vi "Error parser.vi"(0 "Data Readed":string, 11 "error in (no error)":errorcluster) -> (15 "error out":errorcluster)   [LabVIEW 2024, in "GRBL 1.1.lvlib"]
doc: "This Vi transfort error status from GRBL to LabVIEW inteligible error code."
uses:
  GRBL 1.1.lvlib
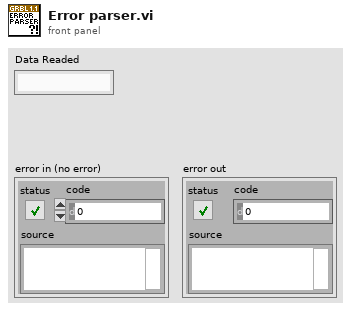
[diagram p1: front panel]
types:
  T1 = cluster{"Code V1.1":i32, "error constant":errorcluster}[]
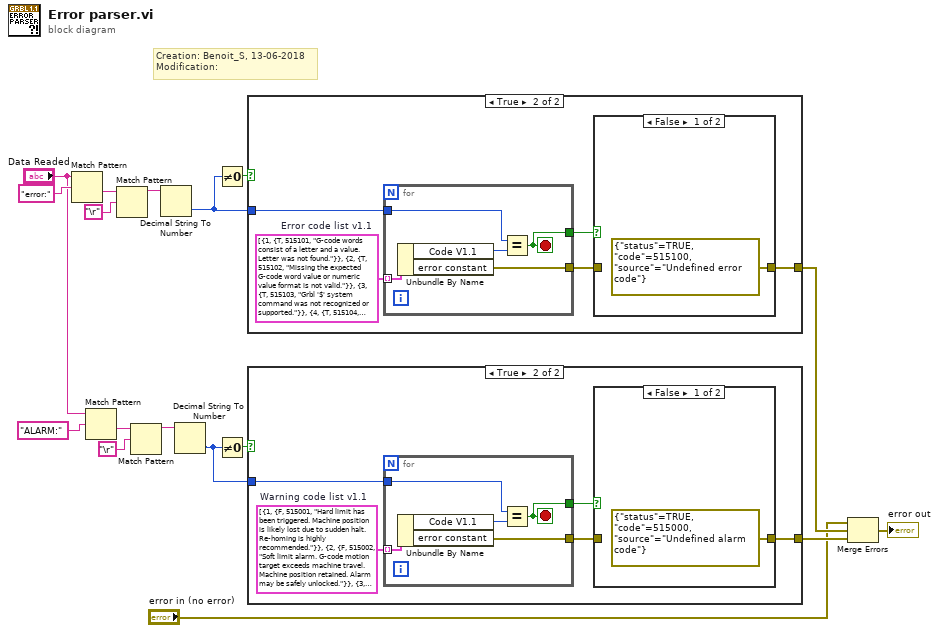
[diagram p0: block diagram]
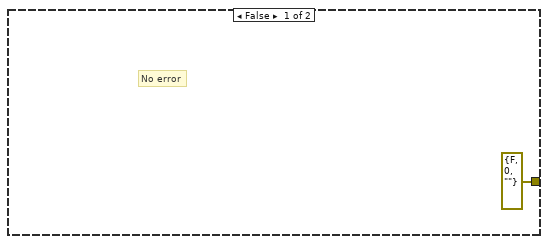
[diagram p2: hidden frame]
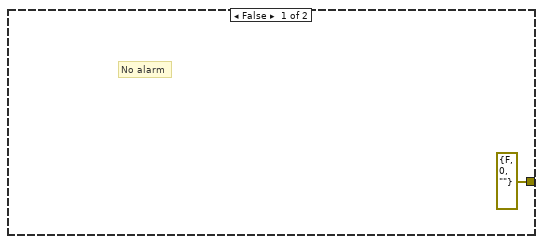
[diagram p4: hidden frame]
diagram:
  # "Creation: Benoit_S, 13-06-2018\nModification:"
  n1 = Match Pattern(string="Data Readed", regular expression="error:") -> (after substring=w10:string)  [unwired: 1 in, 3 out]
  n2 = Match Pattern(string="Data Readed", regular expression="ALARM:") -> (after substring=w4:string)  [unwired: 1 in, 3 out]
  n3 = Match Pattern(string=w10, regular expression="\r") -> (before substring=w8:string)  [unwired: 1 in, 3 out]
  n4 = Match Pattern(string=w4, regular expression="\r") -> (before substring=w6:string)  [unwired: 1 in, 3 out]
  n5 = Decimal String To Number(string=w8) -> (number=w7:i32)  [unwired: 2 in, 1 out]
  n6 = Decimal String To Number(string=w6) -> (number=w3:i32)  [unwired: 2 in, 1 out]
  n7 = Not Equal To 0?(x=w7) -> (x != 0?=w16:bool)
  n8 = Not Equal To 0?(x=w3) -> (x != 0?=w17:bool)
  n9 = case shown="True" w16 {
    tunnel: w7 -> [_ w23]
    tunnel: [errorcluster {"status"=FALSE, "code"=0, "source"=""} ("error constant") w20] -> w14
    frame False {
      # "No error"
    }
    frame True {
      w19 = T1 [{"Code V1.1"=1, "error constant"={"status"=TRUE, "code"=515101, "source"="G-code words consist of a letter and a value. Letter was not found."}}, {"Code V1.1"=2, "error constant"={"status"=TRUE, "code"=515102, "source"="Missing the expected G-code word value or numeric value format is not valid."}}, {"Code V1.1"=3, "error constant"={"status"=TRUE, "code"=515103, "source"="Grbl '$' system command was not recognized or supported."}}, {"Code V1.1"=4, "error constant"={"status"=TRUE, "code"=515104, "source"="Negative value received for an expected positive value."}}, {"Code V1.1"=5, "error constant"={"status"=TRUE, "code"=515105, "source"="Homing cycle failure. Homing is not enabled via settings."}}, {"Code V1.1"=6, "error constant"={"status"=TRUE, "code"=515106, "source"="Minimum step pulse time must be greater than 3usec."}}, {"Code V1.1"=7, "error constant"={"status"=TRUE, "code"=515107, "source"="An EEPROM read failed. Auto-restoring affected EEPROM to default values."}}, {"Code V1.1"=8, "error constant"={"status"=TRUE, "code"=515108, "source"="Grbl '$' command cannot be used unless Grbl is IDLE. Ensures smooth operation during a job."}}, {"Code V1.1"=9, "error constant"={"status"=TRUE, "code"=515109, "source"="G-code commands are locked out during alarm or jog state."}}, {"Code V1.1"=10, "error constant"={"status"=TRUE, "code"=515110, "source"="Soft limits cannot be enabled without homing also enabled."}}, {"Code V1.1"=11, "error constant"={"status"=TRUE, "code"=515111, "source"="Max characters per line exceeded. Received command line was not executed."}}, {"Code V1.1"=12, "error constant"={"status"=TRUE, "code"=515112, "source"="Grbl '$' setting value cause the step rate to exceed the maximum supported."}}, {"Code V1.1"=13, "error constant"={"status"=TRUE, "code"=515113, "source"="Safety door detected as opened and door state initiated."}}, {"Code V1.1"=14, "error constant"={"status"=TRUE, "code"=515114, "source"="Build info or startup line exceeded EEPROM line length limit. Line not stored."}}, {"Code V1.1"=15, "error constant"={"status"=TRUE, "code"=515115, "source"="Jog target exceeds machine travel. Jog command has been ignored."}}, {"Code V1.1"=16, "error constant"={"status"=TRUE, "code"=515116, "source"="Jog command has no '=' or contains prohibited g-code."}}, {"Code V1.1"=17, "error constant"={"status"=TRUE, "code"=515117, "source"="Laser mode requires PWM output."}}, {"Code V1.1"=20, "error constant"={"status"=TRUE, "code"=515120, "source"="Unsupported or invalid g-code command found in block."}}, {"Code V1.1"=21, "error constant"={"status"=TRUE, "code"=515121, "source"="More than one g-code command from same modal group found in block."}}, {"Code V1.1"=22, "error constant"={"status"=TRUE, "code"=515122, "source"="Feed rate has not yet been set or is undefined."}}, {"Code V1.1"=23, "error constant"={"status"=TRUE, "code"=515123, "source"="G-code command in block requires an integer value."}}, {"Code V1.1"=24, "error constant"={"status"=TRUE, "code"=515124, "source"="More than one g-code command that requires axis words found in block."}}, {"Code V1.1"=25, "error constant"={"status"=TRUE, "code"=515125, "source"="Repeated g-code word found in block."}}, {"Code V1.1"=26, "error constant"={"status"=TRUE, "code"=515126, "source"="No axis words found in block for g-code command or current modal state which requires them."}}, {"Code V1.1"=27, "error constant"={"status"=TRUE, "code"=515127, "source"="Line number value is invalid."}}, {"Code V1.1"=28, "error constant"={"status"=TRUE, "code"=515128, "source"="G-code command is missing a required value word."}}, {"Code V1.1"=29, "error constant"={"status"=TRUE, "code"=515129, "source"="G59.x work coordinate systems are not supported."}}, {"Code V1.1"=30, "error constant"={"status"=TRUE, "code"=515130, "source"="G53 only allowed with G0 and G1 motion modes."}}, {"Code V1.1"=31, "error constant"={"status"=TRUE, "code"=515131, "source"="Axis words found in block when no command or current modal state uses them."}}, {"Code V1.1"=32, "error constant"={"status"=TRUE, "code"=515132, "source"="G2 and G3 arcs require at least one in-plane axis word."}}, {"Code V1.1"=33, "error constant"={"status"=TRUE, "code"=515133, "source"="Motion command target is invalid."}}, {"Code V1.1"=34, "error constant"={"status"=TRUE, "code"=515134, "source"="Arc radius value is invalid."}}, {"Code V1.1"=35, "error constant"={"status"=TRUE, "code"=515135, "source"="G2 and G3 arcs require at least one in-plane offset word."}}, {"Code V1.1"=36, "error constant"={"status"=TRUE, "code"=515136, "source"="Unused value words found in block."}}, {"Code V1.1"=37, "error constant"={"status"=TRUE, "code"=515137, "source"="G43.1 dynamic tool length offset is not assigned to configured tool length axis."}}, {"Code V1.1"=38, "error constant"={"status"=TRUE, "code"=515138, "source"="Tool number greater than max supported value."}}]  # Error code list v1.1
      n10 = for {
        tunnel: w19 -> [w30] mode=indexing
        tunnel: w23 -> [w28]
        tunnel: [w27] -> w21
        tunnel: [w26] -> w22
        stop <- w26 stop-if-true
        n11 = Unbundle By Name(w30) -> ("Code V1.1"=w29:i32, "error constant"=w27:errorcluster)
        n12 = Equal?(x=w28, y=w29) -> (x = y?=w26:bool)
      }
      n13 = case shown="False" w22 {
        tunnel: w21 -> [_ w25]
        tunnel: [errorcluster {"status"=TRUE, "code"=515100, "source"="Undefined error code"} ("error constant") w25] -> w20
        frame False {
        }
        frame True {
        }
      }
    }
  }
  n14 = case shown="True" w17 {
    tunnel: w3 -> [_ w35]
    tunnel: [errorcluster {"status"=FALSE, "code"=0, "source"=""} ("error constant") w32] -> w15
    frame False {
      # "No alarm"
    }
    frame True {
      w36 = T1 [{"Code V1.1"=1, "error constant"={"status"=FALSE, "code"=515001, "source"="Hard limit has been triggered. Machine position is likely lost due to sudden halt. Re-homing is highly recommended."}}, {"Code V1.1"=2, "error constant"={"status"=FALSE, "code"=515002, "source"="Soft limit alarm. G-code motion target exceeds machine travel. Machine position retained. Alarm may be safely unlocked."}}, {"Code V1.1"=3, "error constant"={"status"=FALSE, "code"=515003, "source"="Reset while in motion. Machine position is likely lost due to sudden halt. Re-homing is highly recommended."}}, {"Code V1.1"=4, "error constant"={"status"=FALSE, "code"=515004, "source"="Probe fail. Probe is not in the expected initial state before starting probe cycle when G38.2 and G38.3 is not triggered and G38.4 and G38.5 is triggered."}}, {"Code V1.1"=5, "error constant"={"status"=FALSE, "code"=515005, "source"="Probe fail. Probe did not contact the workpiece within the programmed travel for G38.2 and G38.4."}}, {"Code V1.1"=6, "error constant"={"status"=FALSE, "code"=515006, "source"="Homing fail. The active homing cycle was reset."}}, {"Code V1.1"=7, "error constant"={"status"=FALSE, "code"=515007, "source"="Homing fail. Safety door was opened during homing cycle."}}, {"Code V1.1"=8, "error constant"={"status"=FALSE, "code"=515008, "source"="Homing fail. Pull off travel failed to clear limit switch. Try increasing pull-off setting or check wiring."}}, {"Code V1.1"=9, "error constant"={"status"=FALSE, "code"=515009, "source"="Homing fail. Could not find limit switch within search distances. Try increasing max travel"}}]  # Warning code list v1.1
      n15 = for {
        tunnel: w36 -> [w43] mode=indexing
        tunnel: w35 -> [w41]
        tunnel: [w40] -> w33
        tunnel: [w39] -> w34
        stop <- w39 stop-if-true
        n16 = Unbundle By Name(w43) -> ("Code V1.1"=w42:i32, "error constant"=w40:errorcluster)
        n17 = Equal?(x=w41, y=w42) -> (x = y?=w39:bool)
      }
      n18 = case shown="False" w34 {
        tunnel: w33 -> [_ w38]
        tunnel: [errorcluster {"status"=TRUE, "code"=515000, "source"="Undefined alarm code"} ("error constant") w38] -> w32
        frame False {
        }
        frame True {
        }
      }
    }
  }
  n19 = Merge Errors("error in (no error)", w14, w15) -> (→"error out":errorcluster)
